vi "update the test result table.vi"(4 "Step Test":bool, 5 "Step Test Index":i32, 6 "Bool引用句柄":refnum<vi>, 7 "Test Result":string[](array[string]), 8 "数组":string[][](array[string]), 9 "Test Start Time":string, 10 "Test Table":refnum<vi>, 11 "LED":T1) -> ()   [LabVIEW 2016]
uses:
  <vilib>/Utility/miscctls.llb/LVRowAndColumnTypeDef.ctl
  Global Variables/Pacemaker ASIC Test_Save_SN Globals.vi
  Global Variables/Pacemaker ASIC Test_Config Globals.vi
  <vilib>/Utility/file.llb/Write Delimited Spreadsheet (string).vi
panel:
  in  "Test Unit Information":string[][](array[string])=[["Module", "SRN"], ["Software", "V01"]]
  in  "清除原有数据":bool
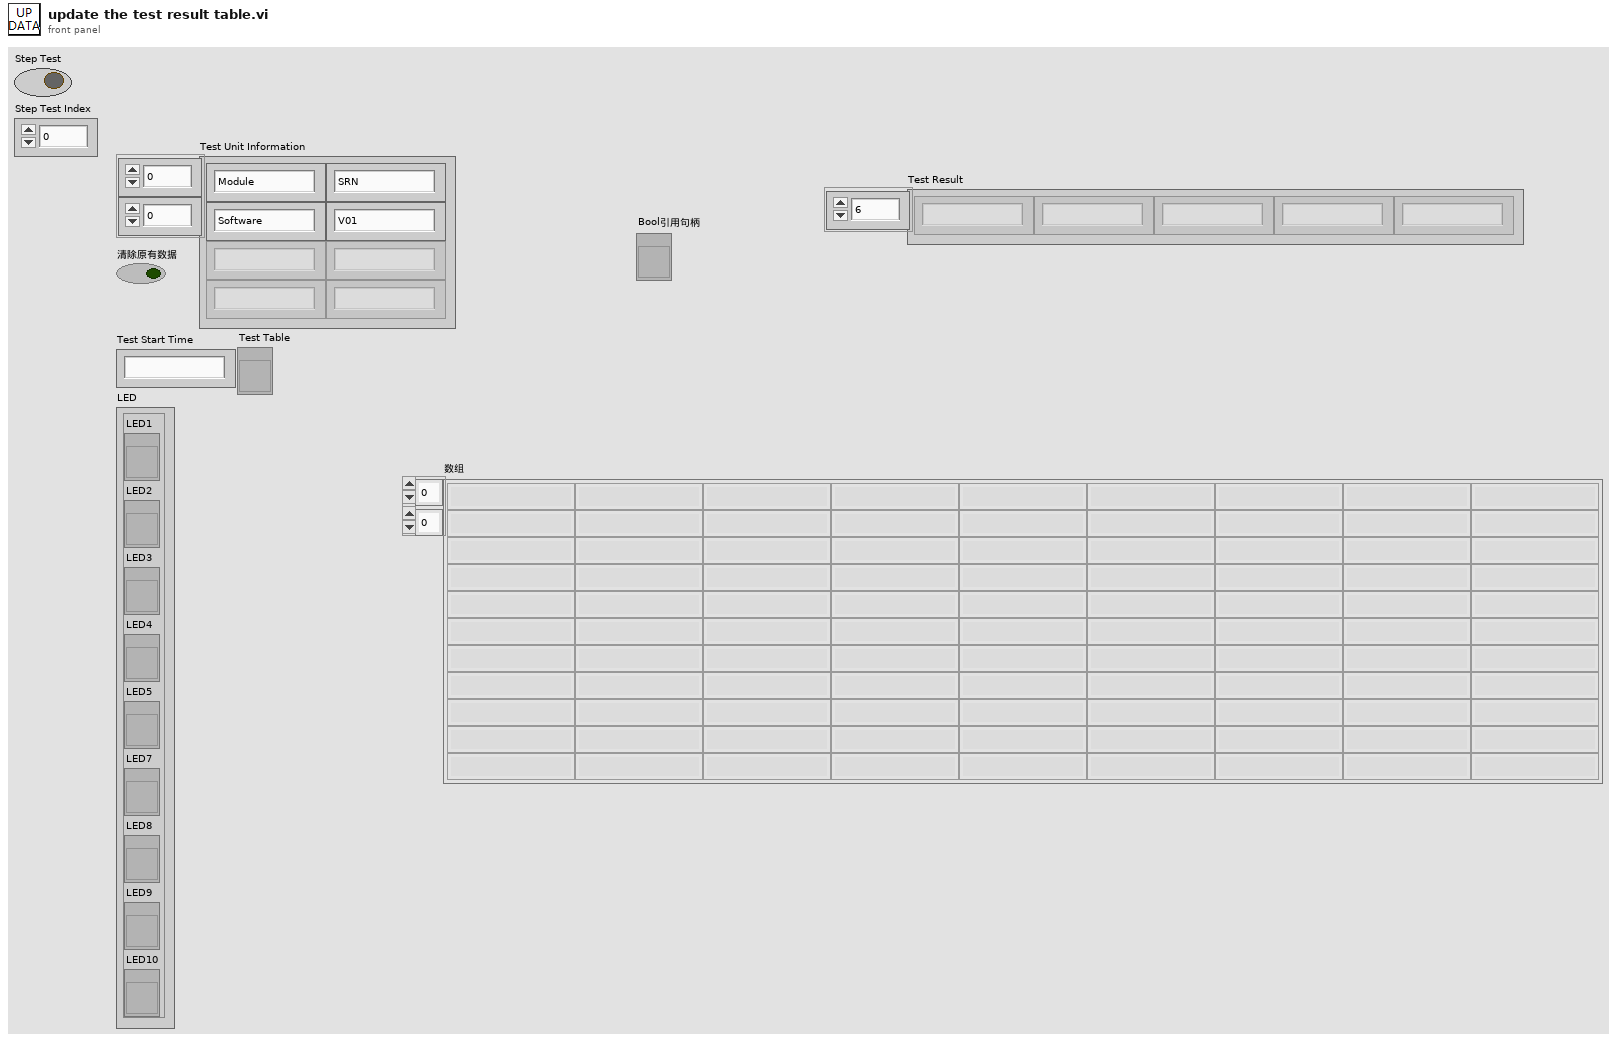
[diagram p1: front panel]
types:
  T1 = cluster{"LED1":refnum<vi>, "LED2":refnum<vi>, "LED3":refnum<vi>, "LED4":refnum<vi>, "LED5":refnum<vi>, "LED7":refnum<vi>, "LED8":refnum<vi>, "LED9":refnum<vi>, "LED10":refnum<vi>}
  T2 = typedef "LVRowAndColumnTypeDef.ctl" = cluster{"Row":i32, "Column":i32}
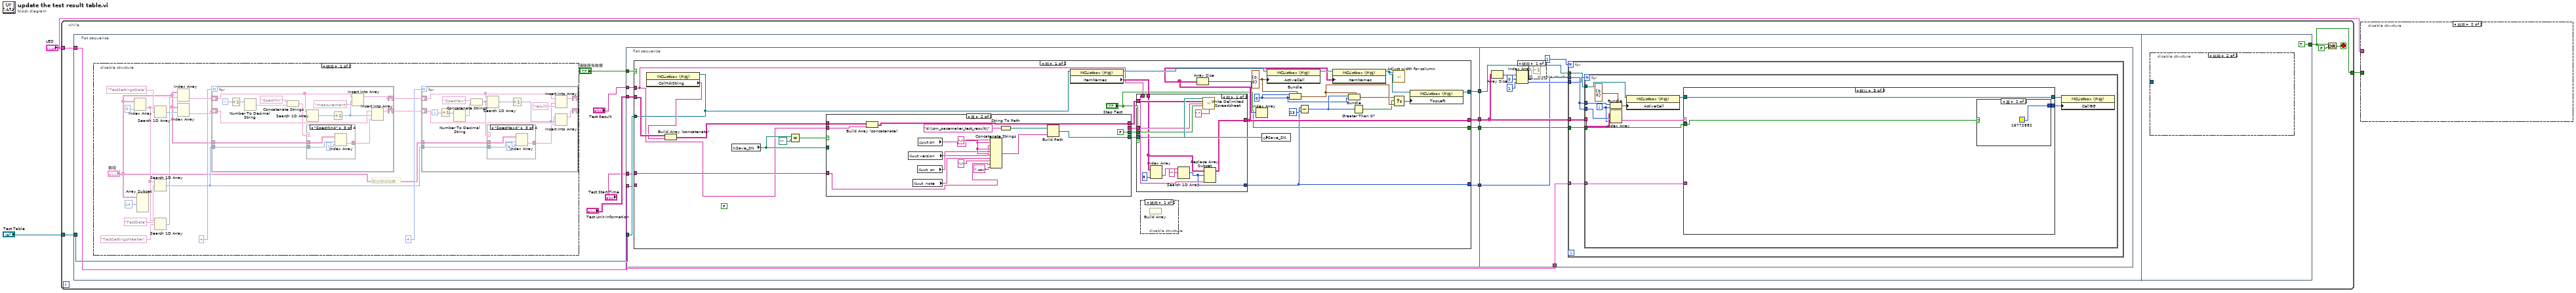
[diagram p0: block diagram]
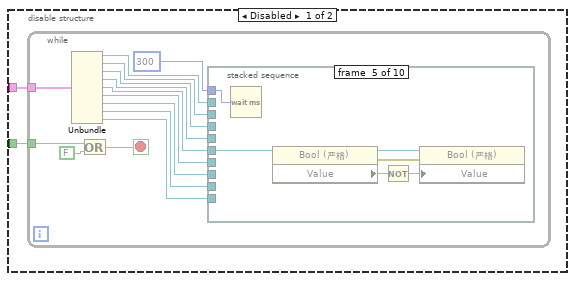
[diagram p2: hidden frame]
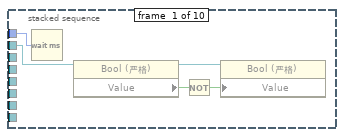
[diagram p3: hidden frame]
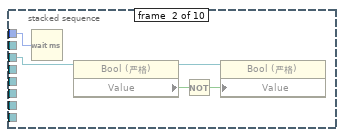
[diagram p4: hidden frame]
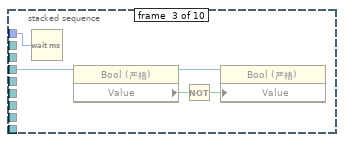
[diagram p5: hidden frame]
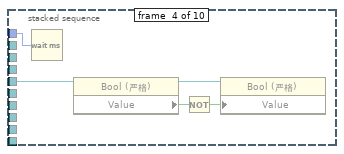
[diagram p6: hidden frame]
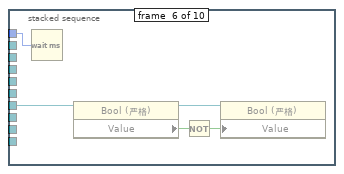
[diagram p7: hidden frame]
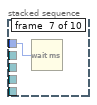
[diagram p8: hidden frame]
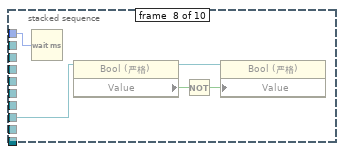
[diagram p9: hidden frame]
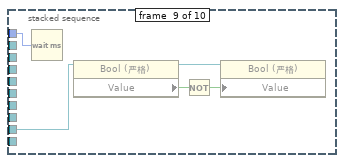
[diagram p10: hidden frame]
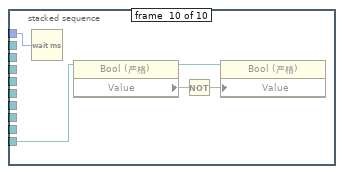
[diagram p11: hidden frame]
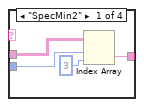
[diagram p12: hidden frame]
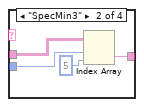
[diagram p13: hidden frame]
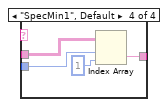
[diagram p14: hidden frame]
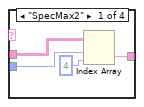
[diagram p15: hidden frame]
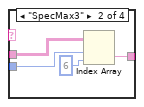
[diagram p16: hidden frame]
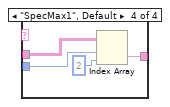
[diagram p17: hidden frame]
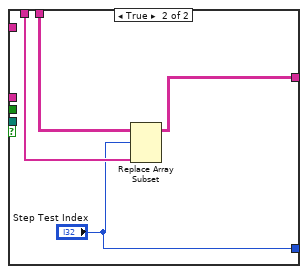
[diagram p19: hidden frame]
diagram:
  n1 = while {
    tunnel: "Test Table" -> [w8]
    tunnel: [w5] -> w3
    tunnel: "LED" -> [w4]
    stop <- w6 stop-if-true
    n2 = flat-sequence {
      tunnel: w8 -> [w15]
      tunnel: w4 -> [w14]
      tunnel: [TRUE] -> w5
      frame #0 {
        n3 = disable-structure shown="禁用" {
          frame Disabled {
            # "取出测试结果"
            n4 = Index Array(array="数组", index (col)=0 ("禁用的索引 (列)")) -> (element=w23:string[])  [unwired: 1 in]
            n5 = Array Subset(array="数组", length (row)=14 ("长度")) -> ()  [unwired: 3 in, 1 out]
            n6 = Search 1D Array(1D array=w23, element="TestSettingsData" ("元素")) -> (index of element=w24:i32)  [unwired: 1 in]
            n7 = Search 1D Array(1D array=w23, element="TestData" ("元素")) -> (index of element=w21:i32)  [unwired: 1 in]
            n8 = Search 1D Array(1D array=w23, element="TestSettingsHeader" ("元素")) -> (index of element=w26:i32)  [unwired: 1 in]
            n9 = Index Array(array="数组", index (row)=w26) -> (element=w34:string[])  [unwired: 1 in]
            n10 = Index Array(array="数组", index (row)=w24) -> (element=w32:string[])  [unwired: 1 in]
            n11 = for {
              N: 4 -> [_]
              shift-right: [w43] -> w31
              shift-left: w34 -> [w44]
              shift-right: [w40] -> w30
              shift-left: w32 -> [w41]
              tunnel: "数组" -> [w36]
              tunnel: w21 -> [w35]
              i -> [w48]
              n12 = Increment(x=w48) -> (x+1=w47:i32)
              n13 = Number To Decimal String(number=w47) -> (decimal integer string=w46:string)  [unwired: 1 in]
              n14 = Concatenate Strings("SpecMin" ("元素"), w46) -> (w45:string)
              n15 = Search 1D Array(1D array=w44, element=w45) -> (index of element=w42:i32)  [unwired: 1 in]
              n16 = case shown="\"SpecMin4\"" w45 {
                tunnel: w36 -> [w52 w56 w58 w65]
                tunnel: [w51 w54 w60 w63] -> w38
                tunnel: w35 -> [w50 w55 w59 w62]
                frame "SpecMin2" {
                  n17 = Index Array(array=w52, index (row)=w50, index (col)=3) -> (element=w51:string)
                }
                frame "SpecMin3" {
                  n18 = Index Array(array=w56, index (row)=w55, index (col)=5) -> (element=w54:string)
                }
                frame "SpecMin4" {
                  n19 = Index Array(array=w58, index (row)=w59, index (col)=7) -> (element=w60:string)
                }
                frame "SpecMin1", Default {
                  n20 = Index Array(array=w65, index (row)=w62, index (col)=1) -> (element=w63:string)
                }
              }
              n21 = Increment(x=w42) -> (x+1=w37:i32)
              n22 = Insert Into Array(array=w44, index=w37, new element="measurement" ("新元素/子数组")) -> (w43:string[])
              n23 = Insert Into Array(array=w41, index=w37, new element=w38) -> (w40:string[])
            }
            n24 = for {
              N: 4 -> [_]
              shift-right: [w74] -> _
              shift-left: w31 -> [w75]
              shift-right: [w71] -> _
              shift-left: w30 -> [w72]
              tunnel: "数组" -> [w67]
              tunnel: w21 -> [w66]
              i -> [w79]
              n25 = Increment(x=w79) -> (x+1=w78:i32)
              n26 = Number To Decimal String(number=w78) -> (decimal integer string=w77:string)  [unwired: 1 in]
              n27 = Concatenate Strings("SpecMax" ("元素"), w77) -> (w76:string)
              n28 = Search 1D Array(1D array=w75, element=w76) -> (index of element=w73:i32)  [unwired: 1 in]
              n29 = case shown="\"SpecMax4\"" w76 {
                tunnel: w67 -> [w83 w87 w90 w96]
                tunnel: [w82 w85 w91 w94] -> w69
                tunnel: w66 -> [w81 w86 w89 w93]
                frame "SpecMax2" {
                  n30 = Index Array(array=w83, index (row)=w81, index (col)=4) -> (element=w82:string)
                }
                frame "SpecMax3" {
                  n31 = Index Array(array=w87, index (row)=w86, index (col)=6) -> (element=w85:string)
                }
                frame "SpecMax4" {
                  n32 = Index Array(array=w90, index (row)=w89, index (col)=8) -> (element=w91:string)
                }
                frame "SpecMax1", Default {
                  n33 = Index Array(array=w96, index (row)=w93, index (col)=2) -> (element=w94:string)
                }
              }
              n34 = Increment(x=w73) -> (x+1=w68:i32)
              n35 = Insert Into Array(array=w75, index=w68, new element="result" ("新元素/子数组")) -> (w74:string[])
              n36 = Insert Into Array(array=w72, index=w68, new element=w69) -> (w71:string[])
            }
          }
          frame Enabled {
          }
        }
        n37 = flat-sequence {
          tunnel: "Test Result" -> [w106]
          tunnel: "清除原有数据" -> [w105]
          tunnel: w15 -> [w104]
          tunnel: [w103] -> w18
          tunnel: [w102] -> w17
          tunnel: w14 -> [w101]
          tunnel: "Test Unit Information" -> [w100]
          tunnel: "Test Start Time" -> [w99]
          tunnel: [w98] -> w10
          tunnel: [w97] -> w9
          tunnel: w18 -> [w259]
          tunnel: w17 -> [w258]
          tunnel: w14 -> [w257]
          tunnel: w10 -> [w254]
          tunnel: w9 -> [w253]
          frame #0 {
            n38 = case shown="假" w105 {
              tunnel: w106 -> [w110 _]
              tunnel: w104 -> [w112 w194]
              tunnel: [w109 _] -> w103
              tunnel: [w120 w192] -> w102
              tunnel: w101 -> [_ w191]
              tunnel: w100 -> [w133 _]
              tunnel: w99 -> [w113 _]
              tunnel: [w108 _] -> w98
              tunnel: ["Step Test" _] -> w97
              frame False {
                (unwired) FALSE
                w115 = 0
                w124 = T2 {"Row"=0, "Column"=0} ("活动单元格:活动单元格")
                n39 = property class="MCListbox (严格)"(reference=w112) -> ("ColHdrString"=w114:string[])  [unwired: 1 in, 2 out]
                n40 = Build Array (concatenate)(w133, w114) -> (w134:string[][])
                n41 = global read "Pacemaker ASIC Test_Save_SN Globals.vi" "Save_SN"() -> (w130:path)
                n42 = Equal?(x=w130, y=path "") -> (x = y?=w131:bool)
                n43 = case shown="真" w131 {
                  tunnel: w134 -> [_ w159]
                  tunnel: w130 -> [w155 _]
                  tunnel: [w155 w161] -> w129
                  tunnel: [_ w157] -> w128
                  tunnel: [TRUE FALSE] -> w127
                  tunnel: w110 -> [w153 w158]
                  tunnel: [w153 _] -> w126
                  tunnel: w113 -> [_ w156]
                  frame False {
                  }
                  frame True {
                    w170 = "-"
                    n44 = Build Array (concatenate)(w159, w158) -> (w157:string[][])
                    n45 = global read "Pacemaker ASIC Test_Config Globals.vi" "uut version"() -> (w168:string)
                    n46 = global read "Pacemaker ASIC Test_Config Globals.vi" "uut  note"() -> (w171:string)
                    n47 = global read "Pacemaker ASIC Test_Config Globals.vi" "uut  sn"() -> (w169:string)
                    n48 = global read "Pacemaker ASIC Test_Config Globals.vi" "uut pn"() -> (w167:string)
                    n49 = Concatenate Strings(w167, w170, w168, w170, w169, w170, w171, "-", w156, ".csv" ("字符串")) -> (w163:string)
                    n50 = String To Path(string="d:\\srn_pacemaker_test_result\\" ("字符串")) -> (path=w164:path)
                    n51 = Build Path(base path=w164, name or relative path=w163) -> (appended path=w161:path)
                  }
                }
                n52 = property class="MCListbox (严格)"(reference=w112) -> (reference out=w135:refnum<vi>, "ItemNames"=w111:string[][])  [unwired: 1 in, 1 out]
                n53 = case shown="假" "Step Test" {
                  tunnel: w129 -> [w148 _]
                  tunnel: w128 -> [w147 _]
                  tunnel: w127 -> [w146 _]
                  tunnel: w126 -> [w145 _]
                  tunnel: w111 -> [w140 w152]
                  tunnel: w110 -> [w139 w151]
                  tunnel: [w138 w150] -> w109
                  tunnel: [w137 "Step Test Index"] -> w108
                  frame False {
                    n54 = Index Array(array=w140, index (col)=8 ("禁用的索引 (列)")) -> (element=w142:string[])  [unwired: 1 in]
                    n55 = Search 1D Array(1D array=w142, element="" ("元素")) -> (index of element=w137:i32)  [unwired: 1 in]
                    n56 = call-poly <vilib>:"Write Delimited Spreadsheet.vi"("file path (dialog if empty)"=w148, "2D data"=w147, "1D data"=w145, "append to file? (new file:F)"=w146, "delimiter (\\t)"="," ("delimiter (\\t)")) -> ()  [unwired: 9 in, 2 out]
                    n57 = Replace Array Subset(array=w140, new element=w139, index (row)=w137) -> (w138:string[][])  [unwired: 1 in]
                  }
                  frame True {
                    n58 = Replace Array Subset(array=w152, new element=w151, index (row)="Step Test Index") -> (w150:string[][])  [unwired: 1 in]
                  }
                }
                n59 = disable-structure shown="禁用" {
                  frame Disabled {
                    n60 = Build Array() -> ()  [unwired: 2 in, 1 out]
                  }
                  frame Enabled {
                  }
                }
                n61 = Array Size(array=w109) -> (size(s)=w125:i32[])
                n62 = Index Array(array=w125) -> ()  [unwired: 1 in, 1 out]
                n63 = global write "Pacemaker ASIC Test_Save_SN Globals.vi" "Save_SN"(w129) -> ()
                n64 = property class="MCListbox (严格)"(reference=w135, "ActiveCell"=w124) -> (reference out=w136:refnum<vi>)  [unwired: 1 in, 1 out]
                n65 = Bundle(cluster=w124, "Row"=w115, "Column"=w115) -> (w123:T2)
                n66 = Subtract(x=w108, y=23) -> (x-y=w116:i32)
                n67 = property class="MCListbox (严格)"(reference=w136, "ItemNames"=w109) -> (reference out=w119:refnum<vi>)  [unwired: 1 in, 1 out]
                n68 = Bundle(cluster=w123, "Row"=w116, "Column"=w115) -> (w122:T2)
                n69 = Greater Than 0?(x=w116) -> (x > 0?=w117:bool)
                n70 = call "Adjust width for column.vi"("MCListbox引用句柄"=w119) -> ()  [unwired: 11 in]
                n71 = Select(t=w122, s=w117, f=w123) -> (s? t:f=w121:T2)
                n72 = property class="MCListbox (严格)"(reference=w119, "TopLeft"=w121) -> (reference out=w120:refnum<vi>)  [unwired: 1 in, 1 out]
              }
              frame True {
                # "初始化MCListbox到空"
                n73 = property class="MCListbox (严格)"(reference=w194, "ActiveCell"=T2 {"Row"=0, "Column"=0} ("活动单元格:活动单元格")) -> (reference out=w179:refnum<vi>)  [unwired: 1 in, 1 out]
                n74 = property class="MCListbox (严格)"(reference=w179) -> (reference out=w178:refnum<vi>, "ItemNames"=w177:string[][])  [unwired: 1 in, 1 out]
                n75 = Array Size(array=w177) -> (size(s)=w176:i32[])
                n76 = property class="MCListbox (严格)"(reference=w178, "ItemNames"=string[][] [] ("项名")) -> (reference out=w193:refnum<vi>)  [unwired: 1 in, 1 out]
                n77 = Index Array(array=w176, index #1=0 ("索引"), index #2=1 ("索引")) -> (element #1=w174:i32, element #2=w172:i32)
                n78 = for {
                  N: w174 -> [_]
                  tunnel: w193 -> [w239]
                  tunnel: [w238] -> w192
                  tunnel: w172 -> [w237]
                  i -> [w240]
                  n79 = for {
                    N: w237 -> [_]
                    tunnel: w240 -> [w247]
                    tunnel: w239 -> [w244]
                    tunnel: [w243] -> w238
                    i -> [w246]
                    n80 = Bundle(cluster=cluster{i32, i32} {0, 0} ("簇"), w247, w246) -> (w248:cluster{i32, i32})
                    n81 = property class="MCListbox (严格)"(reference=w244, "ActiveCell"=w248) -> (reference out=w241:refnum<vi>)  [unwired: 1 in, 1 out]
                    n82 = disable-structure shown="启用" {
                      disable-tunnel: w241 -> [w251 _]
                      disable-tunnel: [w250 _] -> _
                      disable-tunnel: [w249 _] -> _
                      frame Disabled {
                        n83 = property class="MCListbox (严格)"(reference=w251) -> (reference out=w250:refnum<vi>, "CellBG"=w252:u32)  [unwired: 1 in, 1 out]
                        n84 = Not Equal?(x=w252) -> (x != y?=w249:bool)  [unwired: 1 in]
                      }
                      frame Enabled {
                      }
                    }
                    n85 = property class="MCListbox (严格)"(reference=w241, "CellBG"=u32 16448250) -> (reference out=w243:refnum<vi>)  [unwired: 1 in, 1 out]
                  }
                }
                n86 = Unbundle(w191) -> ("LED1"=w190:refnum<vi>, "LED2"=w189:refnum<vi>, "LED3"=w188:refnum<vi>, "LED4"=w187:refnum<vi>, "LED5"=w186:refnum<vi>, "LED7"=w185:refnum<vi>, "LED8"=w182:refnum<vi>, "LED9"=w183:refnum<vi>, "LED10"=w184:refnum<vi>)
                n87 = stacked-sequence {
                  tunnel: w190 -> [w200 _ _ _ _ _ _ _ _ _]
                  tunnel: w189 -> [_ w204 _ _ _ _ _ _ _ _]
                  tunnel: w188 -> [_ _ w208 _ _ _ _ _ _ _]
                  tunnel: w187 -> [_ _ _ w212 _ _ _ _ _ _]
                  tunnel: w186 -> [_ _ _ _ w216 _ _ _ _ _]
                  tunnel: w185 -> [_ _ _ _ _ w220 _ _ _ _]
                  tunnel: w184 -> [_ _ _ _ _ _ _ _ _ w236]
                  tunnel: w183 -> [_ _ _ _ _ _ _ _ w231 _]
                  tunnel: w182 -> [_ _ _ _ _ _ w224 w228 _ _]
                  tunnel: cluster{u32, u32}[] [{1985280, 1985280}, {65358, 65358}, {1985280, 1985280}, {6618880, 6618880}] ("颜色[4]") -> [w199 w203 w207 w211 w215 w219 w223 w227 w232 w235]
                  tunnel: TRUE -> [w198 w202 w206 w209 w213 w217 w221 w225 w229 w233]
                  frame #0 {
                    n88 = property class="Bool (严格)"(reference=w200, "Colors [4]"=w199) -> (reference out=w197:refnum<vi>)  [unwired: 1 in, 1 out]
                    n89 = property class="Bool (严格)"(reference=w197, "Value"=w198) -> ()  [unwired: 1 in, 2 out]
                  }
                  frame #1 {
                    n90 = property class="Bool (严格)"(reference=w204, "Colors [4]"=w203) -> (reference out=w201:refnum<vi>)  [unwired: 1 in, 1 out]
                    n91 = property class="Bool (严格)"(reference=w201, "Value"=w202) -> ()  [unwired: 1 in, 2 out]
                  }
                  frame #2 {
                    n92 = property class="Bool (严格)"(reference=w208, "Colors [4]"=w207) -> (reference out=w205:refnum<vi>)  [unwired: 1 in, 1 out]
                    n93 = property class="Bool (严格)"(reference=w205, "Value"=w206) -> ()  [unwired: 1 in, 2 out]
                  }
                  frame #3 {
                    n94 = property class="Bool (严格)"(reference=w212, "Colors [4]"=w211) -> (reference out=w210:refnum<vi>)  [unwired: 1 in, 1 out]
                    n95 = property class="Bool (严格)"(reference=w210, "Value"=w209) -> ()  [unwired: 1 in, 2 out]
                  }
                  frame #4 {
                    n96 = property class="Bool (严格)"(reference=w216, "Colors [4]"=w215) -> (reference out=w214:refnum<vi>)  [unwired: 1 in, 1 out]
                    n97 = property class="Bool (严格)"(reference=w214, "Value"=w213) -> ()  [unwired: 1 in, 2 out]
                  }
                  frame #5 {
                    n98 = property class="Bool (严格)"(reference=w220, "Colors [4]"=w219) -> (reference out=w218:refnum<vi>)  [unwired: 1 in, 1 out]
                    n99 = property class="Bool (严格)"(reference=w218, "Value"=w217) -> ()  [unwired: 1 in, 2 out]
                  }
                  frame #6 {
                    n100 = property class="Bool (严格)"(reference=w224, "Colors [4]"=w223) -> (reference out=w222:refnum<vi>)  [unwired: 1 in, 1 out]
                    n101 = property class="Bool (严格)"(reference=w222, "Value"=w221) -> ()  [unwired: 1 in, 2 out]
                  }
                  frame #7 {
                    n102 = property class="Bool (严格)"(reference=w228, "Colors [4]"=w227) -> (reference out=w226:refnum<vi>)  [unwired: 1 in, 1 out]
                    n103 = property class="Bool (严格)"(reference=w226, "Value"=w225) -> ()  [unwired: 1 in, 2 out]
                  }
                  frame #8 {
                    n104 = property class="Bool (严格)"(reference=w231, "Colors [4]"=w232) -> (reference out=w230:refnum<vi>)  [unwired: 1 in, 1 out]
                    n105 = property class="Bool (严格)"(reference=w230, "Value"=w229) -> ()  [unwired: 1 in, 2 out]
                  }
                  frame #9 {
                    n106 = property class="Bool (严格)"(reference=w236, "Colors [4]"=w235) -> (reference out=w234:refnum<vi>)  [unwired: 1 in, 1 out]
                    n107 = property class="Bool (严格)"(reference=w234, "Value"=w233) -> ()  [unwired: 1 in, 2 out]
                  }
                }
              }
            }
          }
          frame #1 {
            n108 = Array Size(array=w259) -> (size(s)=w263:i32[])
            n109 = Index Array(array=w263, index #1=0 ("索引"), index #2=1 ("索引")) -> (element #1=w256:i32, element #2=w260:i32)
            n110 = disable-structure shown="禁用" {
              disable-tunnel: w256 -> [w264 _]
              frame Disabled {
                n111 = Decrement(x=w264) -> ()  [unwired: 1 out]
              }
              frame Enabled {
              }
            }
            n112 = for {
              N: 1 -> [_]
              tunnel: w260 -> [w270]
              tunnel: w259 -> [w269]
              tunnel: w258 -> [w268]
              tunnel: w257 -> [w267]
              tunnel: w254 -> [w266]
              tunnel: w253 -> [w265]
              n113 = for {
                N: w270 -> [_]
                tunnel: w266 -> [w283]
                tunnel: w269 -> [w282]
                tunnel: w266 -> [w279]
                tunnel: w268 -> [w273]
                tunnel: w267 -> [w272]
                tunnel: w265 -> [w271]
                i -> [w278]
                n114 = Bundle(cluster=cluster{i32, i32} {0, 0} ("簇"), w279, w278) -> (w280:cluster{i32, i32})
                n115 = Index Array(array=w282, index (row)=w283, index (col)=w278) -> (element=w281:string)
                n116 = property class="MCListbox (严格)"(reference=w273, "ActiveCell"=w280) -> (reference out=w277:refnum<vi>)  [unwired: 1 in, 1 out]
                n117 = case shown="默认" w281 {
                  tunnel: w277 -> [w285 w291 w347]
                  tunnel: [w285 w291 w347] -> w276
                  tunnel: [u32 6618880 u32 16711680 w346] -> w274
                  tunnel: w272 -> [_ w289 _]
                  tunnel: w271 -> [_ w286 w345]
                  frame "Pass" {
                  }
                  frame "Fail" {
                    n118 = case shown="假" w286 {
                      frame False {
                        n119 = global read "Pacemaker ASIC Test_Save_SN Globals.vi" "Save_SN"() -> (w292:path)
                        n120 = Path To String(path=w292) -> (string=w294:string)
                        n121 = Search and Replace String(input string=w294, search string="Fail" ("搜索字符串")) -> (offset past replacement=w297:i32)  [unwired: 6 in, 3 out]
                        n122 = Equal?(x=w297, y=-1) -> (x = y?=w295:bool)
                        n123 = case shown="真" w295 {
                          tunnel: w294 -> [_ w303]
                          tunnel: [w299 w306] -> w293
                          tunnel: w292 -> [w299 w307]
                          frame False {
                          }
                          frame True {
                            n124 = Search and Replace String(input string=w303, search string="." ("搜索字符串"), replace string="_Fail." ("字符串")) -> (result string=w300:string)  [unwired: 5 in, 3 out]
                            n125 = String To Path(string=w300) -> (path=w306:path)
                            n126 = flat-sequence {
                              tunnel: w307 -> [w309]
                              tunnel: w306 -> [w310]
                              tunnel: [w309] -> w304
                              tunnel: [w311] -> w305
                              tunnel: w304 -> [w311]
                              tunnel: w305 -> [w313]
                              frame #0 {
                                n127 = Copy(9:TRUE ("覆盖(F)"), 10:w310, 11:w309) -> ()  [unwired: 2 in, 3 out]
                              }
                              frame #1 {
                                n128 = Wait (ms)(milliseconds to wait=u32 100 ("等待时间（毫秒）")) -> ()  [unwired: 1 out]
                              }
                              frame #2 {
                                n129 = Delete(path (use dialog)=w313) -> ()  [unwired: 4 in, 3 out]
                              }
                            }
                          }
                        }
                        n130 = global write "Pacemaker ASIC Test_Save_SN Globals.vi" "Save_SN"(w293) -> ()
                      }
                      frame True {
                      }
                    }
                    n131 = disable-structure shown="禁用" {
                      disable-tunnel: w289 -> [w315 _]
                      frame Disabled {
                        n132 = Unbundle(w315) -> ("LED1"=w324:refnum<vi>, "LED2"=w323:refnum<vi>, "LED3"=w322:refnum<vi>, "LED4"=w321:refnum<vi>, "LED5"=w320:refnum<vi>, "LED7"=w319:refnum<vi>, "LED8"=w316:refnum<vi>, "LED9"=w317:refnum<vi>, "LED10"=w318:refnum<vi>)
                        n133 = stacked-sequence {
                          tunnel: w324 -> [w326 _ _ _ _ _ _ _ _ _]
                          tunnel: w323 -> [_ w328 _ _ _ _ _ _ _ _]
                          tunnel: w322 -> [_ _ w330 _ _ _ _ _ _ _]
                          tunnel: w321 -> [_ _ _ w332 _ _ _ _ _ _]
                          tunnel: w320 -> [_ _ _ _ w334 _ _ _ _ _]
                          tunnel: w319 -> [_ _ _ _ _ w336 _ _ _ _]
                          tunnel: w318 -> [_ _ _ _ _ _ _ _ _ w344]
                          tunnel: w317 -> [_ _ _ _ _ _ _ _ w341 _]
                          tunnel: w316 -> [_ _ _ _ _ _ w338 w340 _ _]
                          tunnel: cluster{u32, u32}[] [{1985280, 1985280}, {16711680, 16711680}, {1985280, 1985280}, {6618880, 6618880}] ("颜色[4]") -> [w325 w327 w329 w331 w333 w335 w337 w339 w342 w343]
                          frame #0 {
                            n134 = property class="Bool (严格)"(reference=w326, "Colors [4]"=w325) -> ()  [unwired: 1 in, 2 out]
                          }
                          frame #1 {
                            n135 = property class="Bool (严格)"(reference=w328, "Colors [4]"=w327) -> ()  [unwired: 1 in, 2 out]
                          }
                          frame #2 {
                            n136 = property class="Bool (严格)"(reference=w330, "Colors [4]"=w329) -> ()  [unwired: 1 in, 2 out]
                          }
                          frame #3 {
                            n137 = property class="Bool (严格)"(reference=w332, "Colors [4]"=w331) -> ()  [unwired: 1 in, 2 out]
                          }
                          frame #4 {
                            n138 = property class="Bool (严格)"(reference=w334, "Colors [4]"=w333) -> ()  [unwired: 1 in, 2 out]
                          }
                          frame #5 {
                            n139 = property class="Bool (严格)"(reference=w336, "Colors [4]"=w335) -> ()  [unwired: 1 in, 2 out]
                          }
                          frame #6 {
                            n140 = property class="Bool (严格)"(reference=w338, "Colors [4]"=w337) -> ()  [unwired: 1 in, 2 out]
                          }
                          frame #7 {
                            n141 = property class="Bool (严格)"(reference=w340, "Colors [4]"=w339) -> ()  [unwired: 1 in, 2 out]
                          }
                          frame #8 {
                            n142 = property class="Bool (严格)"(reference=w341, "Colors [4]"=w342) -> ()  [unwired: 1 in, 2 out]
                          }
                          frame #9 {
                            n143 = property class="Bool (严格)"(reference=w344, "Colors [4]"=w343) -> ()  [unwired: 1 in, 2 out]
                          }
                        }
                      }
                      frame Enabled {
                      }
                    }
                    n144 = property class="Bool (严格)"(reference="Bool引用句柄", "Value"=TRUE ("值")) -> ()  [unwired: 1 in, 2 out]
                  }
                  frame Default {
                    n145 = case shown="真" w345 {
                      tunnel: [u32 16448250 u32 16772882] -> w346
                      frame False {
                      }
                      frame True {
                      }
                    }
                  }
                }
                n146 = property class="MCListbox (严格)"(reference=w276, "CellBG"=w274) -> ()  [unwired: 1 in, 2 out]
              }
            }
          }
        }
      }
      frame #1 {
        n147 = disable-structure shown="启用" {
          disable-tunnel: _ -> [w351 _]
          frame Disabled {
            n148 = stacked-sequence {
              tunnel: w351 -> [w357 w363]
              tunnel: 100 -> [w354 w360]
              tunnel: [_ w359] -> w352
              frame #0 {
                w356 = TRUE
                n149 = Wait (ms)(milliseconds to wait=w354) -> ()  [unwired: 1 out]
                n150 = Variant To Data(type=w356, Variant=w356) -> (data=w355:bool)  [unwired: 1 in, 1 out]
                n151 = invoke class="VI (严格)" method="Ctrl Val.Set"(reference=w357, "Control Name"="Blinking" ("控件名"), "Value"=w355) -> ()  [unwired: 2 in, 5 out]
              }
              frame #1 {
                w362 = FALSE
                n152 = Wait (ms)(milliseconds to wait=w360) -> ()  [unwired: 1 out]
                n153 = Variant To Data(type=w362, Variant=w362) -> (data=w361:bool)  [unwired: 1 in, 1 out]
                n154 = invoke class="VI (严格)" method="Ctrl Val.Set"(reference=w363, "Control Name"="Blinking" ("控件名"), "Value"=w361) -> (reference out=w359:refnum<vi>)  [unwired: 2 in, 4 out]
              }
            }
            n155 = Close Reference(reference=w352) -> ()  [unwired: 1 in, 1 out]
          }
          frame Enabled {
          }
        }
      }
    }
    n156 = Or(x=w5, y=FALSE) -> (x .or. y?=w6:bool)
  }
  n157 = disable-structure shown="启用" {
    disable-tunnel: w3 -> [w366 _]
    disable-tunnel: "LED" -> [w365 _]
    frame Disabled {
      n158 = while {
        tunnel: w365 -> [w380]
        tunnel: w366 -> [w369]
        stop <- w368 stop-if-true
        n159 = Unbundle(w380) -> ("LED1"=w379:refnum<vi>, "LED2"=w377:refnum<vi>, "LED3"=w376:refnum<vi>, "LED4"=w375:refnum<vi>, "LED5"=w374:refnum<vi>, "LED7"=w373:refnum<vi>, "LED8"=w370:refnum<vi>, "LED9"=w371:refnum<vi>, "LED10"=w372:refnum<vi>)
        n160 = Or(x=w369, y=FALSE) -> (x .or. y?=w368:bool)
        n161 = stacked-sequence {
          tunnel: w379 -> [w385 _ _ _ _ _ _ _ _ _]
          tunnel: 300 -> [w381 w388 w391 w396 w402 w409 w412 w415 w418 w425]
          tunnel: w377 -> [_ w390 _ _ _ _ _ _ _ _]
          tunnel: w376 -> [_ _ w392 _ _ _ _ _ _ _]
          tunnel: w375 -> [_ _ _ w400 _ _ _ _ _ _]
          tunnel: w374 -> [_ _ _ _ w401 _ _ _ _ _]
          tunnel: w373 -> [_ _ _ _ _ w408 _ _ _ _]
          tunnel: w372 -> [_ _ _ _ _ _ _ _ _ w427]
          tunnel: w371 -> [_ _ _ _ _ _ _ _ w422 _]
          tunnel: w370 -> [_ _ _ _ _ _ _ w417 _ _]
          frame #0 {
            n162 = Wait (ms)(milliseconds to wait=w381) -> ()  [unwired: 1 out]
            n163 = property class="Bool (严格)"(reference=w385) -> (reference out=w384:refnum<vi>, "Value"=w383:bool)  [unwired: 1 in, 1 out]
            n164 = Not(x=w383) -> (.not. x?=w382:bool)
            n165 = property class="Bool (严格)"(reference=w384, "Value"=w382) -> ()  [unwired: 1 in, 2 out]
          }
          frame #1 {
            n166 = Wait (ms)(milliseconds to wait=w388) -> ()  [unwired: 1 out]
            n167 = property class="Bool (严格)"(reference=w390) -> (reference out=w389:refnum<vi>, "Value"=w387:bool)  [unwired: 1 in, 1 out]
            n168 = Not(x=w387) -> (.not. x?=w386:bool)
            n169 = property class="Bool (严格)"(reference=w389, "Value"=w386) -> ()  [unwired: 1 in, 2 out]
          }
          frame #2 {
            n170 = Wait (ms)(milliseconds to wait=w391) -> ()  [unwired: 1 out]
            n171 = property class="Bool (严格)"(reference=w392) -> (reference out=w393:refnum<vi>, "Value"=w395:bool)  [unwired: 1 in, 1 out]
            n172 = Not(x=w395) -> (.not. x?=w394:bool)
            n173 = property class="Bool (严格)"(reference=w393, "Value"=w394) -> ()  [unwired: 1 in, 2 out]
          }
          frame #3 {
            n174 = Wait (ms)(milliseconds to wait=w396) -> ()  [unwired: 1 out]
            n175 = property class="Bool (严格)"(reference=w400) -> (reference out=w399:refnum<vi>, "Value"=w398:bool)  [unwired: 1 in, 1 out]
            n176 = Not(x=w398) -> (.not. x?=w397:bool)
            n177 = property class="Bool (严格)"(reference=w399, "Value"=w397) -> ()  [unwired: 1 in, 2 out]
          }
          frame #4 {
            n178 = Wait (ms)(milliseconds to wait=w402) -> ()  [unwired: 1 out]
            n179 = property class="Bool (严格)"(reference=w401) -> (reference out=w406:refnum<vi>, error out=w405:errorcluster, "Value"=w404:bool)  [unwired: 1 in]
            n180 = Not(x=w404) -> (.not. x?=w403:bool)
            n181 = property class="Bool (严格)"(reference=w406, error in=w405, "Value"=w403) -> ()  [unwired: 2 out]
          }
          frame #5 {
            n182 = Wait (ms)(milliseconds to wait=w409) -> ()  [unwired: 1 out]
            n183 = property class="Bool (严格)"(reference=w408) -> (reference out=w407:refnum<vi>, "Value"=w411:bool)  [unwired: 1 in, 1 out]
            n184 = Not(x=w411) -> (.not. x?=w410:bool)
            n185 = property class="Bool (严格)"(reference=w407, "Value"=w410) -> ()  [unwired: 1 in, 2 out]
          }
          frame #6 {
            n186 = Wait (ms)(milliseconds to wait=w412) -> ()  [unwired: 1 out]
          }
          frame #7 {
            n187 = Wait (ms)(milliseconds to wait=w415) -> ()  [unwired: 1 out]
            n188 = property class="Bool (严格)"(reference=w417) -> (reference out=w416:refnum<vi>, "Value"=w414:bool)  [unwired: 1 in, 1 out]
            n189 = Not(x=w414) -> (.not. x?=w413:bool)
            n190 = property class="Bool (严格)"(reference=w416, "Value"=w413) -> ()  [unwired: 1 in, 2 out]
          }
          frame #8 {
            n191 = Wait (ms)(milliseconds to wait=w418) -> ()  [unwired: 1 out]
            n192 = property class="Bool (严格)"(reference=w422) -> (reference out=w421:refnum<vi>, "Value"=w420:bool)  [unwired: 1 in, 1 out]
            n193 = Not(x=w420) -> (.not. x?=w419:bool)
            n194 = property class="Bool (严格)"(reference=w421, "Value"=w419) -> ()  [unwired: 1 in, 2 out]
          }
          frame #9 {
            n195 = Wait (ms)(milliseconds to wait=w425) -> ()  [unwired: 1 out]
            n196 = property class="Bool (严格)"(reference=w427) -> (reference out=w426:refnum<vi>, "Value"=w424:bool)  [unwired: 1 in, 1 out]
            n197 = Not(x=w424) -> (.not. x?=w423:bool)
            n198 = property class="Bool (严格)"(reference=w426, "Value"=w423) -> ()  [unwired: 1 in, 2 out]
          }
        }
      }
    }
    frame Enabled {
    }
  }
